vi "ToDo-2018-03-23.vi"() -> ()   [LabVIEW 2019]
uses:
  SMOs/DAQ_Manager/DAQ_Manager.lvclass
  SMOs/DAQmx.AO/Typedefs/AO.Terminal-enum.ctl
  SMOs/DAQmx.AO/DAQmx.AO.lvclass
  SMOs/DAQmx.AO/Typedefs/DAQmx.AO_Config.ctl
  SMOs/DAQmx.AI/Typedefs/AI.Terminal-enum.ctl
  SMOs/DAQmx.AI/DAQmx.AI.lvclass
  SMOs/DAQmx.AI/Typedefs/AI.Coupling-enum.ctl
  SMOs/DAQmx.AI/Typedefs/DAQmx.AI_Config.ctl
  SMOs/DAQ_Manager/Typedefs/PrivateEvents--DAQ_Manager.setDAQConfig.ctl
  SMOs/UI_DAQ_config/UI_DAQ_config.lvclass
  SMOs/DSP/DSP.lvclass
  SMOs/Generator/Generator.lvclass
  SMOs/UI_DAQ_config/Typedefs/446xAO-enum.ctl
  SMOs/UI_DAQ_config/Typedefs/AO.config-cluster.ctl
  SMOs/UI_DAQ_config/Typedefs/AO.config-array.ctl
  SMOs/UI_DAQ_config/Typedefs/AI.coupling-enum.ctl
  SMOs/UI_DAQ_config/Typedefs/446xAI-enum.ctl
  SMOs/UI_DAQ_config/Typedefs/AI.config-cluster.ctl
  SMOs/UI_DAQ_config/Typedefs/AI.config-array.ctl
panel:
  in  "AI Configuration":T1=[{"AI.Coupling"=enum."AC", "AI.Range"=enum."±0.316 V", "DAQmx Physical Channel"="PXI1Slot2/ai0:1"}, {"AI.Coupling"=enum."AC", "AI.Range"=enum."±0.316 V", "DAQmx Physical Channel"="PXI1Slot3/ai0:1"}, {"AI.Coupling"=enum."AC", "AI.Range"=enum."±0.316 V", "DAQmx Physical Channel"="PXI1Slot4/ai0:1"}, {"AI.Coupling"=enum."AC", "AI.Range"=enum."±0.316 V", "DAQmx Physical Channel"="PXI1Slot5/ai0:1"}]
  in  "AO Configuration":T5=[{"AO.Range"=enum."±0.1 V", "DAQmx Physical Channel"="PXI1Slot2/ao0:1"}, {"AO.Range"=enum."±0.1 V", "DAQmx Physical Channel"="PXI1Slot3/ao0:1"}, {"AO.Range"=enum."±0.1 V", "DAQmx Physical Channel"="PXI1Slot4/ao0:1"}, {"AO.Range"=enum."±0.1 V", "DAQmx Physical Channel"="PXI1Slot5/ao0:1"}]
  in  "SamplingInfo":cluster{"Fs":dbl, "#S":i32}={"Fs"=10000.0, "#S"=1000}
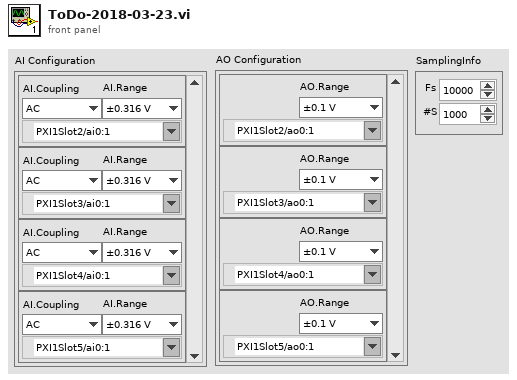
[diagram p1: front panel]
types:
  T1 = typedef "UI_DAQ_config.lvclass/AI.config-array.ctl" = T2[]
  T2 = typedef "UI_DAQ_config.lvclass/AI.config-cluster.ctl" = cluster{"AI.Coupling":T3, "AI.Range":T4, "DAQmx Physical Channel":tag}
  T3 = typedef "UI_DAQ_config.lvclass/AI.coupling-enum.ctl" = enum16{"AC", "DC"}
  T4 = typedef "UI_DAQ_config.lvclass/446xAI-enum.ctl" = enum16{"±0.316 V", "±1.00 V", "±3.16 V", "±10.0 V", "±31.6 V", "±42.4 V"}
  T5 = typedef "UI_DAQ_config.lvclass/AO.config-array.ctl" = T6[]
  T6 = typedef "UI_DAQ_config.lvclass/AO.config-cluster.ctl" = cluster{"AO.Range":T7, "DAQmx Physical Channel":tag}
  T7 = typedef "UI_DAQ_config.lvclass/446xAO-enum.ctl" = enum16{"±0.1 V", "±1.0 V", "±10.0 V"}
  T8 = typedef "DAQ_Manager.lvclass/PrivateEvents--DAQ_Manager.setDAQConfig.ctl" = cluster{"DAQ.Config (AI)":cluster{"Channels":string, "DAQ_Type":enum16{"AI", "AO"}, "minimum value":dbl, "maximum value":dbl, "DAQ_SamplingInfo":cluster{"Fs":dbl, "#s":i32}, "DAQ_SamplingMode":enum16{"Continuous", "Finite"}}[], "DAQmx.AI.config":T9[], "DAQ.Config (AO)":cluster{"Channels":string, "DAQ_Type":enum16{"AI", "AO"}, "minimum value":dbl, "maximum value":dbl, "DAQ_SamplingInfo":cluster{"Fs":dbl, "#s":i32}, "DAQ_SamplingMode":enum16{"Continuous", "Finite"}}[], "DAQmx.AO.config":T12[]}
  T9 = typedef "DAQmx.AI.lvclass/DAQmx.AI_Config.ctl" = cluster{"AI.Coupling":T10, "input terminal configuration ":T11}
  T10 = typedef "DAQmx.AI.lvclass/AI.Coupling-enum.ctl" = i32
  T11 = typedef "DAQmx.AI.lvclass/AI.Terminal-enum.ctl" = i32
  T12 = typedef "DAQmx.AO.lvclass/DAQmx.AO_Config.ctl" = cluster{"output terminal configuration":T13}
  T13 = typedef "DAQmx.AO.lvclass/AO.Terminal-enum.ctl" = i32
  T14 = typedef "DSP.lvclass/PrivateEvents--DSP.RunCalculation.ctl" = cluster{"runCalculation":cluster{"adjust gain":bool, "subtract offset":bool, "60 Hz prefilter":bool, "LP prefilter":bool, "lockin":bool, "FFT":bool, "gain":dbl[], "offset":dbl[], "LP config":T15, "Lockin config":T16, "FFT config":T17}}
  T15 = typedef "DSP.lvclass/LP_Config.ctl" = cluster{"high cutoff freq [Hz]":dbl}
  T16 = typedef "DSP_lockin.lvclass/Lockin_Config.ctl" = cluster{" f (Hz)":dbl, "phi (deg)":dbl, "TC (s)":dbl, "order":i32}[]
  T17 = typedef "DSP.lvclass/FFT_Config.ctl" = cluster{"averaging parameters":cluster{"averaging mode":enum16{"No averaging", "Vector averaging", "RMS averaging", "Peak hold"}, "weighting mode":enum16{"Linear", "Exponential"}, "number of averages":u32}, "window":T18, "export mode":T19, "window parameter":dbl, "restart averaging (F)":bool}
  T18 = typedef "NI_AALPro.lvlib/windowTd.ctl" = u32
  T19 = typedef "NI_MAPro.lvlib/Power Spectrum and PSD Export Mode.ctl" = u16
  T20 = typedef "Generator.lvclass/PrivateEvents--Generator.configGenerator.ctl" = cluster{"A (V)":dbl, "DC (V)":dbl, "f (Hz)":dbl, "phi (deg)":dbl, "signal type":enum16{"Sine Wave", "Triangle Wave", "Square Wave", "Sawtooth Wave"}}[]
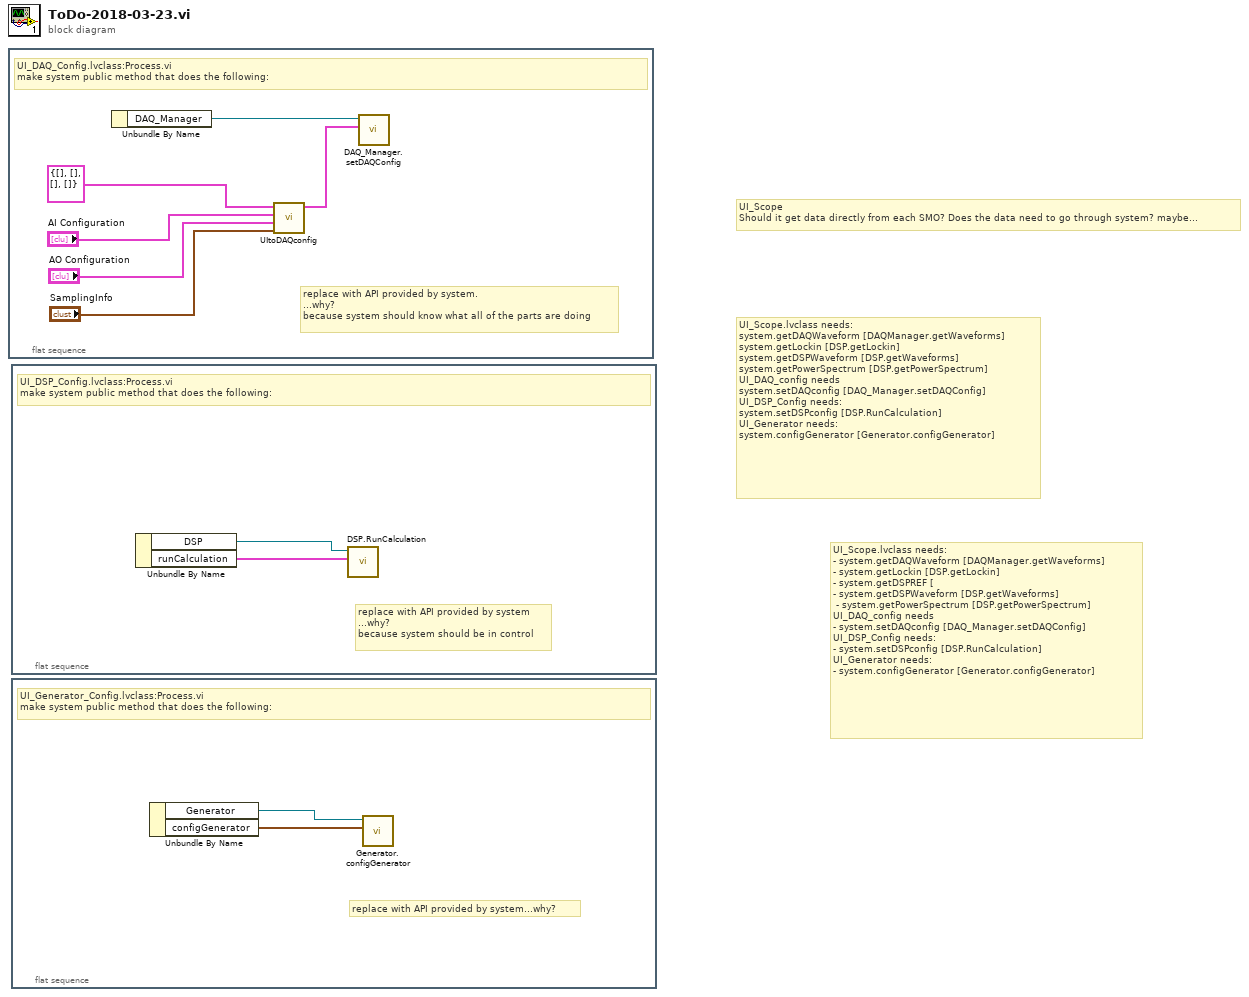
[diagram p0: block diagram]
diagram:
  # "UI_Scope.lvclass needs:\n- system.getDAQWaveform [DAQManager.getWaveforms]\n- system.getLockin [DSP.getLockin]\n- system.getDSPREF [\n- system.getDSPWaveform [DSP.getWaveforms]\n - system.getPowerSpectrum [DSP.getPowerSpectrum]\nUI_DAQ_config needs\n- system.setDAQconfig [DAQ_Manager.setDAQConfig]\nUI_DSP_Config needs:\n- system.setDSPconfig [DSP.RunCalculation]\nUI_Generator needs:\n- system.configGenerator [Generator.configGenerator]"
  # "UI_Scope.lvclass needs:\nsystem.getDAQWaveform [DAQManager.getWaveforms]\nsystem.getLockin [DSP.getLockin]\nsystem.getDSPWaveform [DSP.getWaveforms]\nsystem.getPowerSpectrum [DSP.getPowerSpectrum]\nUI_DAQ_config needs\nsystem.setDAQconfig [DAQ_Manager.setDAQConfig]\nUI_DSP_Config needs:\nsystem.setDSPconfig [DSP.RunCalculation]\nUI_Generator needs:\nsystem.configGenerator [Generator.configGenerator]"
  # "UI_Scope\nShould it get data directly from each SMO? Does the data need to go through system? maybe..."
  n1 = flat-sequence {
    frame #0 {
      # "replace with API provided by system.\n...why?\nbecause system should know what all of the parts are doing"
      # "UI_DAQ_Config.lvclass:Process.vi\nmake system public method that does the following:"
      n2 = Unbundle By Name() -> ("DAQ_Manager"=w1:refnum<class "DAQ_Manager.lvclass">)  [unwired: 1 in]
      n3 = call "UItoDAQconfig.vi"("SamplingInfo"="SamplingInfo", "AO Configuration"="AO Configuration", "AI Configuration"="AI Configuration", "DAQ_Manager.setDAQConfig"=T8 {"DAQ.Config (AI)"=[], "DAQmx.AI.config"=[], "DAQ.Config (AO)"=[], "DAQmx.AO.config"=[]}) -> ("DAQ_Manager.setDAQConfig"=w3:T8)  [unwired: 7 in]
      n4 = call "DAQ_Manager.setDAQConfig.vi"("DAQ_Manager.setDAQConfig"=w3, "DAQ_Manager"=w1) -> ()  [unwired: 8 in, 2 out]
    }
  }
  n5 = flat-sequence {
    frame #0 {
      # "replace with API provided by system\n...why?\nbecause system should be in control"
      # "UI_DSP_Config.lvclass:Process.vi\nmake system public method that does the following:"
      n6 = Unbundle By Name() -> ("DSP"=w8:refnum<class "DSP.lvclass">, "runCalculation"=w7:T14)  [unwired: 1 in]
      n7 = call "DSP.RunCalculation.vi"("runCalculation"=w7, "DSP"=w8) -> ()  [unwired: 8 in, 2 out]
    }
  }
  n8 = flat-sequence {
    frame #0 {
      # "replace with API provided by system...why?"
      # "UI_Generator_Config.lvclass:Process.vi\nmake system public method that does the following:"
      n9 = Unbundle By Name() -> ("Generator"=w10:refnum<class "Generator.lvclass">, "configGenerator"=w9:T20)  [unwired: 1 in]
      n10 = call "Generator.configGenerator.vi"("configGenerator"=w9, "Generator"=w10) -> ()  [unwired: 8 in, 2 out]
    }
  }
